vi "Laser Damage Scan.vi"() -> ()   [LabVIEW 2020]
uses:
  <vilib>/Utility/miscctls.llb/LVPointTypeDef.ctl
  Hardware Configuration/Hardware Configuration Controls/Device Type.ctl
  Hardware Configuration/Hardware Configuration Controls/Device Function.ctl
panel:
  out "Laser Emission":bool
  in  "Laser Settings":bool
  in  "Current Exposure Time (s)":dbl=1.0 max=100.0
  out "Error":bool
  out "Exposure Active":bool
  in  "Timed":bool
  in  "Live":bool
  in  "Scan Rate (Hz)":dbl=1.0 max=100.0
  in  "Total Exposure Time (s)":dbl=1.0 max=100.0
  in  "Laser Power (%)":u8=1 max=100
  in  "Quit":bool
  in  "Calling VI Ref":refnum<vi>
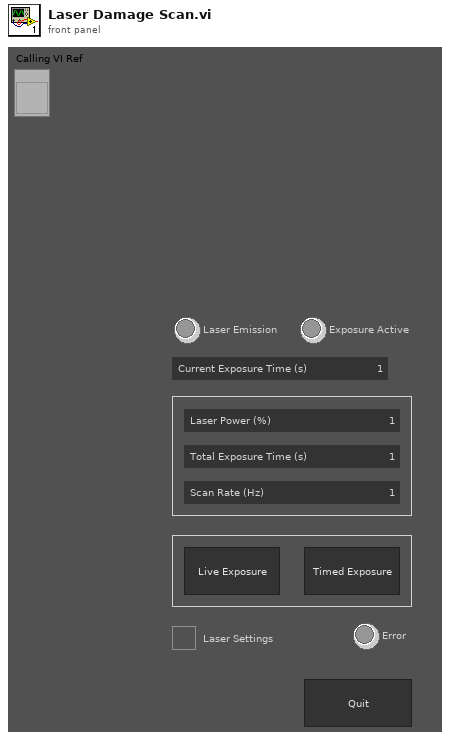
[diagram p1: front panel]
types:
  T1 = typedef "Device Function.ctl" = enum16{"Primary", "Secondary", "Overview", "Wide Field Drift Correction", "642 nm Excitation", "560 nm Excitation", "940 nm Excitation", "546 nm Excitation", "488 nm Excitation", "405 nm Excitation", "Objective Drift Correction", "4Pi Objective Lock", "Objective XY", "Objective Z", "Sample XY", "Sample Coarse Z", "Sample Z", "4Pi Lower", "4Pi Upper", "Mojo", "Adj Cavity", "Line Scanning", "Alert"}
  T2 = typedef "Device Type.ctl" = enum16{"AOTF", "Camera", "Deformable Mirror", "Laser", "Shutter", "Stage", "Waveform", "FPGA", "Email", "Filter Wheel", "Spinning Disk"}
  T3 = enum16{"Always On", "Always Off", "Off While Running"}
  T4 = typedef "LVPointTypeDef.ctl" = cluster{"Horizontal":i16, "Vertical":i16}
  T5 = typedef "LVRectTypeDef.ctl" = cluster{"Left":i16, "Top":i16, "Right":i16, "Bottom":i16}
  T6 = typedef "LVBoundsTypeDef.ctl" = cluster{"Width":u32, "Height":u32}
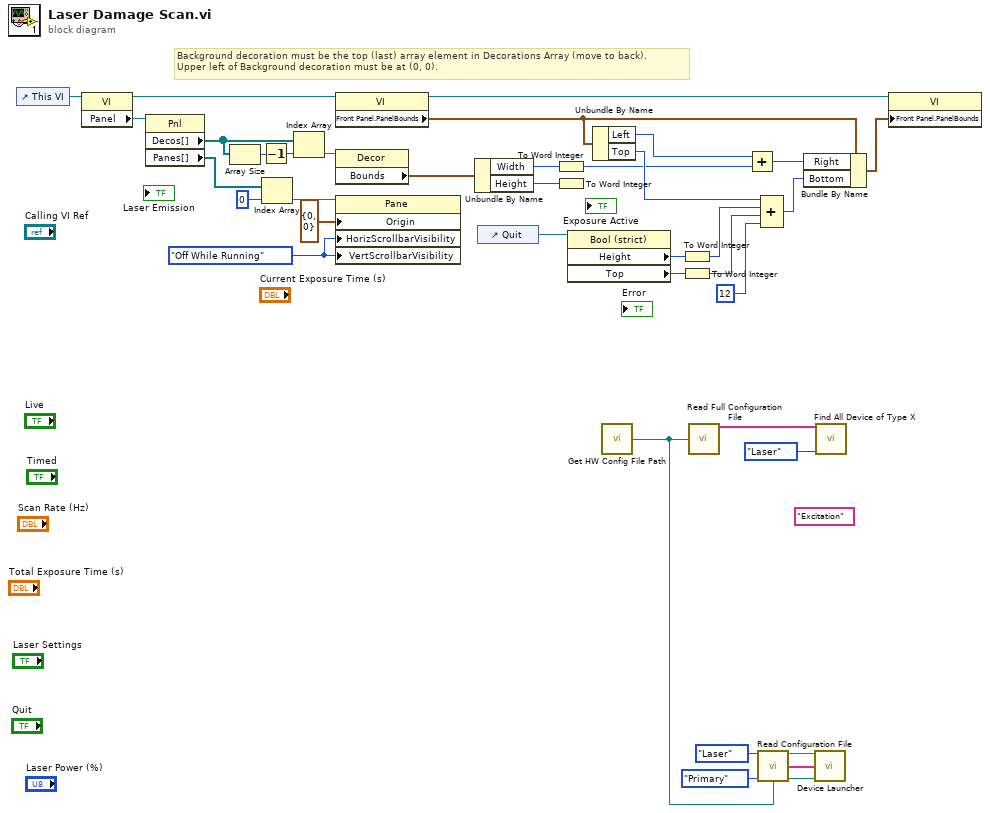
[diagram p0: block diagram]
diagram:
  (unwired) "Excitation"
  w20 = T3."Off While Running" ("Vertical Scrollbar Visibility")
  # "Background decoration must be the top (last) array element in Decorations Array (move to back).\nUpper left of Background decoration must be at (0, 0)."
  n1 = control-ref of="This VI"() -> (w12:refnum<vi>)
  n2 = property class="VI"(reference=w12) -> (reference out=w21:refnum<vi>, "Panel"=w13:refnum<vi>)  [unwired: 1 in, 1 out]
  n3 = property class="Pnl"(reference=w13) -> ("Decos[]"=w11:refnum<vi>[], "Panes[]"=w17:refnum<vi>[])  [unwired: 1 in, 2 out]
  n4 = Array Size(array=w11) -> (size(s)=w9:i32)
  n5 = Decrement(x=w9) -> (x-1=w10:i32)
  n6 = Index Array(array=w17, index=0) -> (element=w16:refnum<vi>)
  n7 = Index Array(array=w11, index=w10) -> (element=w19:refnum<vi>)
  n8 = property class="VI"(reference=w21) -> (reference out=w23:refnum<vi>, "Front Panel.PanelBounds"=w24:T5)  [unwired: 1 in, 1 out]
  n9 = property class="Decor"(reference=w19) -> ("Bounds"=w22:T6)  [unwired: 1 in, 2 out]
  n10 = property class="Pane"(reference=w16, "Origin"=T4 {"Horizontal"=0, "Vertical"=0}, "HorizScrollbarVisibility"=w20, "VertScrollbarVisibility"=w20) -> ()  [unwired: 1 in, 2 out]
  n11 = Unbundle By Name(w22) -> ("Width"=w27:u32, "Height"=w30:u32)
  n12 = control-ref of="Quit"() -> (w14:refnum<vi>)
  n13 = To Word Integer(number=w27) -> (16bit integer=w29:i16)
  n14 = To Word Integer(number=w30) -> ()  [unwired: 1 out]
  n15 = property class="Bool (strict)"(reference=w14) -> ("Height"=w32:u32, "Top"=w33:i32)  [unwired: 1 in, 2 out]
  n16 = Unbundle By Name(w24) -> ("Left"=w26:i16, "Top"=w37:i16)
  n17 = call "Get HW Config File Path.vi"() -> ("File Path"=w4:path)  [unwired: 14 in, 1 out]
  n18 = To Word Integer(number=w32) -> (16bit integer=w35:i16)
  n19 = To Word Integer(number=w33) -> (16bit integer=w36:i16)
  n20 = call "Read Full Configuration File.vi"("Config File Path"=w4) -> ("Unique Notifier Names"=w8:string[])  [unwired: 11 in, 3 out]
  n21 = Add(x=w26, y=w29) -> (x+y=w28:i16)
  n22 = call "Read Configuration File.vi"("Device Type"=Device_Type."Laser", "Device Function"=Device_Function."Primary", "Config File Path"=w4) -> ("Unique Notifier Name"=w3:string, "Device Ports/IDs/Channels"=w2:string[], "Device Engine Path"=w1:path)  [unwired: 9 in, 1 out]
  n23 = Compound Arithmetic op=ADD(w37, w35, w36, i16 12 ("y")) -> (w31:i16)
  n24 = Bundle By Name(cluster=w24, "Right"=w28, "Bottom"=w31) -> (w25:T5)
  n25 = call "Device Launcher.vi"("Notifier Name"=w3, "Device Ports/IDs/Channels"=w2, "Device Engine Path"=w1) -> ()  [unwired: 11 in, 2 out]
  n26 = call "Find All Device of Type X.vi"("Unique Notifier Names"=w8, "Device Type"=Device_Type."Laser") -> ()  [unwired: 12 in, 2 out]
  n27 = property class="VI"(reference=w23, "Front Panel.PanelBounds"=w25) -> ()  [unwired: 1 in, 2 out]
